vi "Process.vi"(8 "error in (no error)":errorcluster, 11 "Process In":refnum<class "Process.lvclass">) -> (0 "error out":errorcluster, 3 "Process Out":refnum<class "Process.lvclass">)   [LabVIEW 2020, in "Process.lvclass"]
uses:
  Process.lvclass
  Process.lvclass/Process.ctl
  <vilib>/ErrorRing/Error Ring.xnode
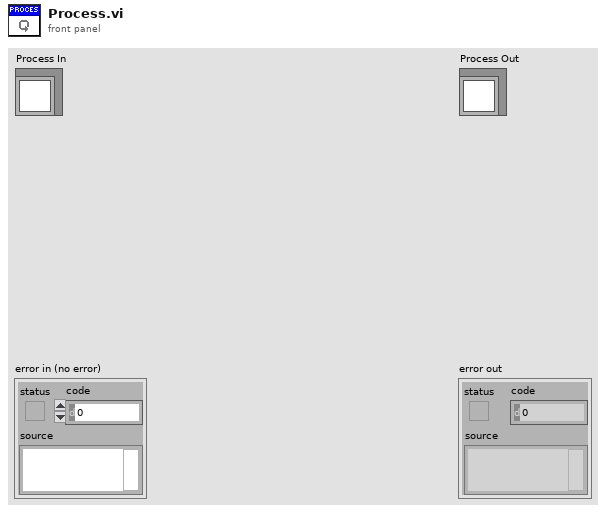
[diagram p1: front panel]
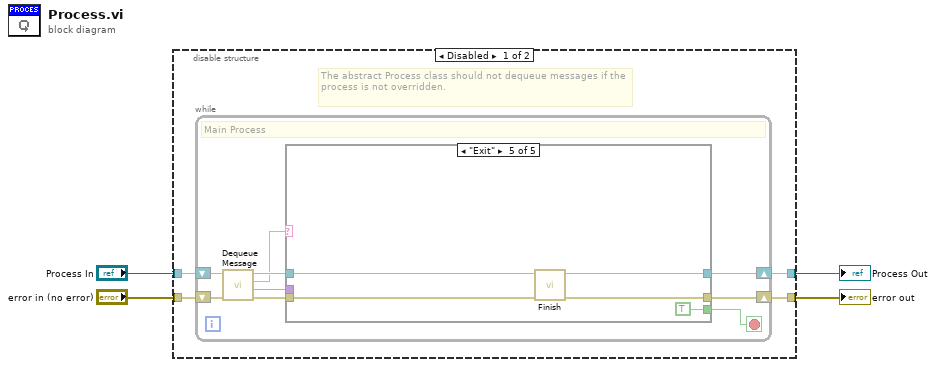
[diagram p0: block diagram]
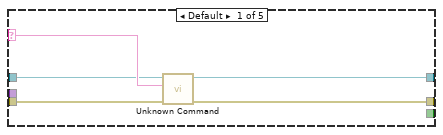
[diagram p2: hidden frame]
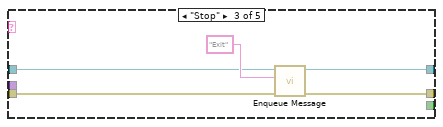
[diagram p4: hidden frame]
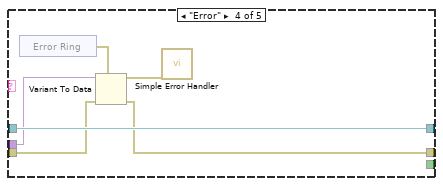
[diagram p5: hidden frame]
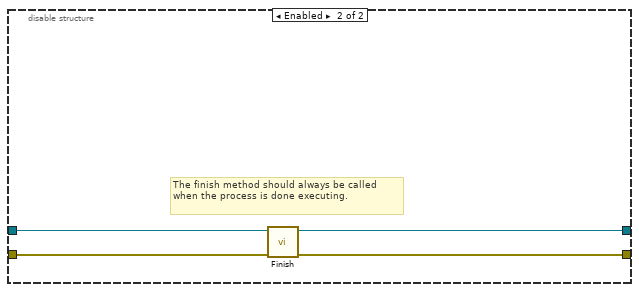
[diagram p6: hidden frame]
diagram:
  n1 = disable-structure shown="Disabled" {
    disable-tunnel: "Process In" -> [w8 w42]
    disable-tunnel: [w7 w43] -> w3
    disable-tunnel: "error in (no error)" -> [w6 w44]
    disable-tunnel: [w5 w45] -> w1
    frame Disabled {
      # "The abstract Process class should not dequeue messages if the process is not overridden."
      n2 = while {
        shift-right: [w12] -> w5
        shift-left: w6 -> [w16]
        shift-right: [w14] -> w7
        shift-left: w8 -> [w17]
        stop <- w9 stop-if-true
        # "Main Process"
        n3 = call "Dequeue Message.vi"("error in (no error)"=w16, "Process In"=w17) -> ("error out"=w15:errorcluster, "Message Data"=w10:variant, "Message"=w11:string, "Process Out"=w13:refnum<class "Process.lvclass">)  [unwired: 6 in]
        n4 = case shown="\"Exit\"" w11 {
          selector: w11 -> [w22 _ _ _ _]
          tunnel: [w19 w23 w26 w31 w38] -> w12
          tunnel: w15 -> [w18 w23 w27 w34 w37]
          tunnel: [w21 w24 w25 w35 w39] -> w14
          tunnel: w13 -> [w20 w24 w28 w35 w40]
          tunnel: w10 -> [_ _ _ w33 _]
          tunnel: [_ _ _ _ TRUE] -> w9
          frame Default {
            n5 = call "Unknown Command.vi"("error in (no error)"=w18, "String"=w22, "Process In"=w20) -> ("error out"=w19:errorcluster, "Process Out"=w21:refnum<class "Process.lvclass">)  [unwired: 7 in]
          }
          frame "Init" {
          }
          frame "Stop" {
            n6 = call "Enqueue Message.vi"("error in (no error)"=w27, "Message"="Exit", "Process In"=w28) -> ("error out"=w26:errorcluster, "Process Out"=w25:refnum<class "Process.lvclass">)  [unwired: 7 in]
          }
          frame "Error" {
            n7 = xnode "Error Ring"() -> ("error out"=w32:errorcluster)
            n8 = Variant To Data(error in=w34, type=w32, Variant=w33) -> (data=w30:errorcluster, error out=w31:errorcluster)
            n9 = call <vilib>:"Simple Error Handler.vi"("error in (no error)"=w30) -> ()  [unwired: 4 in, 5 out]
          }
          frame "Exit" {
            n10 = call "Finish.vi"("error in (no error)"=w37, "Process In"=w40) -> ("error out"=w38:errorcluster, "Process Out"=w39:refnum<class "Process.lvclass">)  [unwired: 8 in]
          }
        }
      }
    }
    frame Enabled {
      # "The finish method should always be called when the process is done executing."
      n11 = call "Finish.vi"("error in (no error)"=w44, "Process In"=w42) -> ("error out"=w45:errorcluster, "Process Out"=w43:refnum<class "Process.lvclass">)  [unwired: 8 in]
    }
  }
  "error out" <- w1
  "Process Out" <- w3
